vi "Send_Multiple.vi"(8 "Error in":errorcluster, 9 "Data":variant[](array[variant]), 10 "Commands":string[](array[string]), 11 "Queue_in":refnum<queue>) -> (0 "Error out":errorcluster, 3 "Queue_out":refnum<queue>)   [LabVIEW 2021]
doc: "Sends multiple commands to the Queue specified in Queue in.\nOptional: Sends data to pe parsed with variant to data to specified cases."
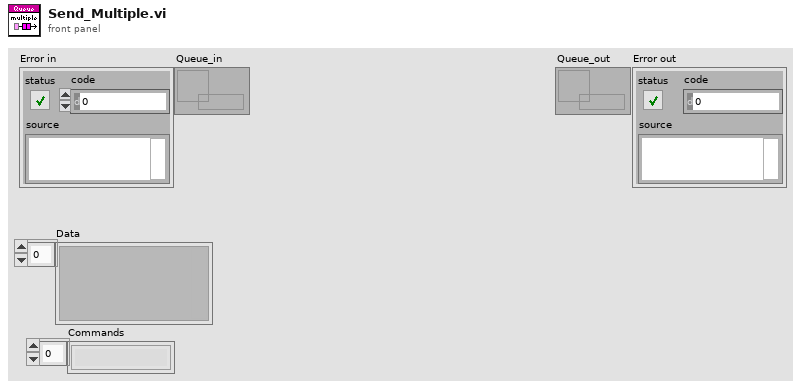
[diagram p1: front panel]
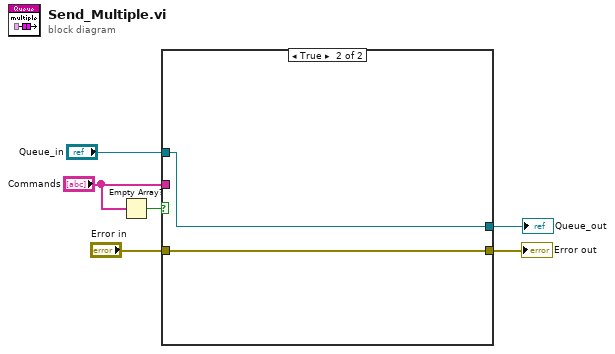
[diagram p0: block diagram]
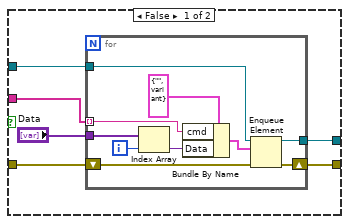
[diagram p2: hidden frame]
diagram:
  n1 = Empty Array?(array="Commands") -> (empty?=w5:bool)
  n2 = case shown="True" w5 {
    tunnel: "Commands" -> [w11 _]
    tunnel: "Error in" -> [w10 w23]
    tunnel: [w9 w23] -> w3
    tunnel: [w8 w24] -> w2
    tunnel: "Queue_in" -> [w7 w24]
    frame False {
      n3 = for {
        tunnel: w7 -> [w22]
        tunnel: w11 -> [w18] mode=indexing
        tunnel: "Data" -> [w21]
        tunnel: [w15] -> w8
        shift-right: [w14] -> w9
        shift-left: w10 -> [w13]
        i -> [w20]
        n4 = Index Array(array=w21, index=w20) -> (element=w17:variant)
        n5 = Bundle By Name(cluster=cluster{"cmd":string, "Data":variant} {"cmd"="", "Data"=variant} ("element"), "cmd"=w18, "Data"=w17) -> (w16:cluster{"cmd":string, "Data":variant})
        n6 = Enqueue Element(queue=w22, element=w16, error in (no error)=w13) -> (queue out=w15:refnum<queue>, error out=w14:errorcluster)  [unwired: 1 in, 1 out]
      }
    }
    frame True {
    }
  }
  "Error out" <- w3
  "Queue_out" <- w2
